vi "String_PadWithCharacters.vi"(5 "char (ASCII)":u8 format="%02x", 7 "length":i32=32, 11 "str in":string) -> (3 "str (padded)":string)   [LabVIEW 2014, in "hse-misc.lvlib"]
doc: "Adds <b>char (ASCII)</b> characters to <b>str in</b> until it is <b>length</b> characters long.\n\nCommon ASCII characters:\n0x09 ... tab\n0x20 ... space\n0x2E ... dot (.)\n____\nHAMPEL SOFTWARE ENGINEERING v0.12.0 (2018-09-13 18:21)"
uses:
  hse-misc.lvlib
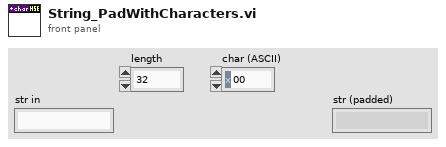
[diagram p1: front panel]
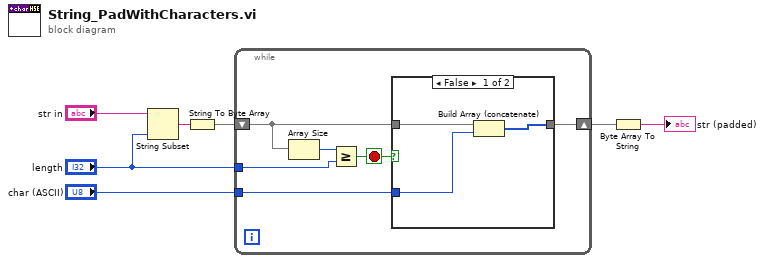
[diagram p0: block diagram]
diagram:
  n1 = String Subset(string="str in", length (rest)="length") -> (substring=w3:string)  [unwired: 1 in]
  n2 = String To Byte Array(string=w3) -> (unsigned byte array=w6:u8[])
  n3 = while {
    shift-right: [w11] -> w7
    shift-left: w6 -> [w12]
    tunnel: "length" -> [w9]
    tunnel: "char (ASCII)" -> [w8]
    stop <- w10 stop-if-true
    n4 = Array Size(array=w12) -> (size(s)=w13:i32)
    n5 = Greater Or Equal?(x=w13, y=w9) -> (x >= y?=w10:bool)
    n6 = case shown="False" w10 {
      tunnel: w12 -> [w16 w17]
      tunnel: [w15 w17] -> w11
      tunnel: w8 -> [w14 _]
      frame False {
        n7 = Build Array (concatenate)(w16, w14) -> (w15:u8[])
      }
      frame True {
      }
    }
  }
  n8 = Byte Array To String(unsigned byte array=w7) -> (string=→"str (padded)":string)
